vi "Que_Parse State.vi"(0 "State Queue":string, 7 "Error In (no error)":errorcluster) -> (4 "Remaining States":string, 6 "Current State":string, 8 "Arguments":string, 10 "PreState":string)   [LabVIEW 2016]
doc: "Parses the JKI State Machine state queue and returns the current state that will execute next with the associated arguments.\n\nFor instructions on how to use the JKI State Machine, examples and video tutorials, visit:\nhttp://jkisoft.com/state-machine/\n\n<B>Inputs:</B>\n <B>State Queue:</B> The entire state queue is wired to this input. This should come from the main JKI State Machine shift register.\n <B>Error In</B> The error cluster from the JKI State Machine is wired to this input. If an error occures and appears on this input, the current state output returns the \"Error Handler\" state.\n\n<B>Outputs:</B>\n <B>Remaining States:</B> Returns all the next states that should execute after the current state completes. These should be passed through the current state in the state machine. These can also be modified or augmented within the current state if necessary.\n <B>Current State:</B> Returns the current state that should execute next in the state machine. If an error is wired to the Error input then the current state output becomes \"Error Handler\".\n <B>Arguments:</B> Returns any argument(s) that may be used in the current state string. These arguments come after the \">>\" characters. <B>Note:</B> The arguments variable must not contain any unprintable characters like linefeed or carriage return.\n\n<B>State Syntax:</B>\nStateCategory: State >> Argument\nLine Terminator: Line feed\n <B>Example:</B>\nUI: Help >> About\n\nWhere \"UI\" is the state category\nWhere \"Help\" is the state\nWhere \"About\" is the argument\n <B>Other Examples:</B>\nApp Data: Initialize\nUI: Initialize\nHelp >> About\n\n<B>Commenting:</B>\nTo add a comment use \"//\" or \"#\" and all text to the right will be ignored\n <B>Commenting Example:</B>\nUI: Initialize // This initializes the UI\n# This whole line is a comment\n// Another comment line\n\nJKI State Machine™\nhttp://jkisoft.com/state-machine/\nCopyright (C) 2005-2008, JKI <info@jkisoft.com>\nALL RIGHTS RESERVED"
panel:
  # "For instructions on how to use the JKI State Machine, examples and video tutorials, visit:\nhttp://jkisoft.com/state-machine/\n\nJKI State Machine™\nhttp://jkisoft.com/state-machine/\nCopyright (C) 2005-2008, JKI <info@jkisoft.com>\nALL RIGHTS RESERVED"
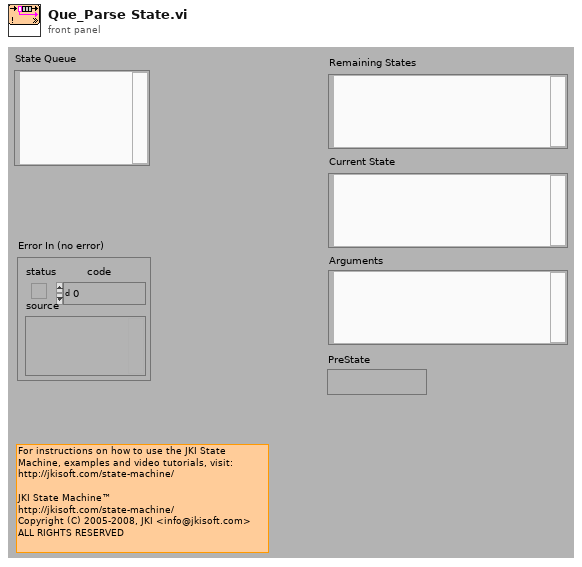
[diagram p1: front panel]
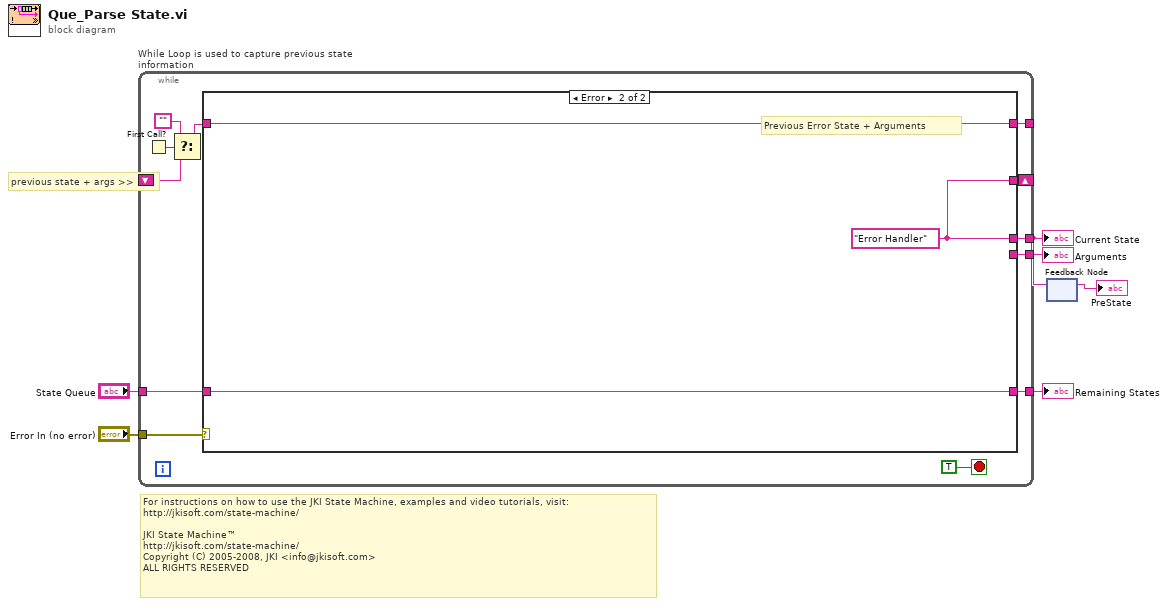
[diagram p0: block diagram]
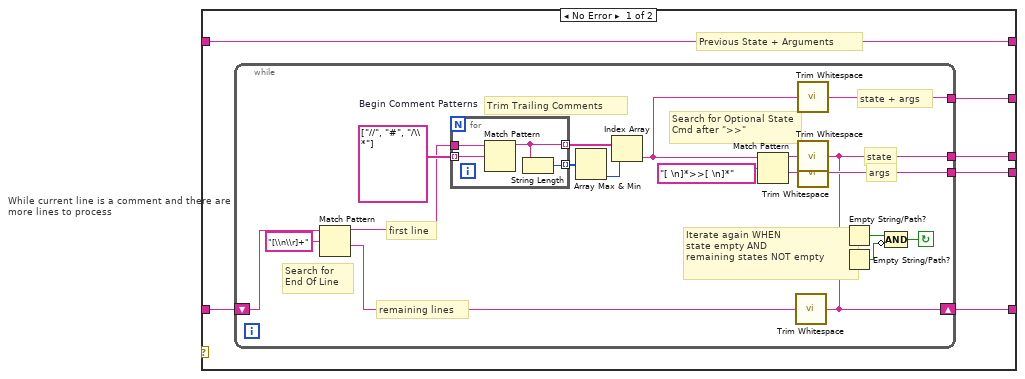
[diagram p2: hidden frame]
diagram:
  # "previous state + args >>"
  # "For instructions on how to use the JKI State Machine, examples and video tutorials, visit:\nhttp://jkisoft.com/state-machine/\n\nJKI State Machine™\nhttp://jkisoft.com/state-machine/\nCopyright (C) 2005-2008, JKI <info@jkisoft.com>\nALL RIGHTS RESERVED"
  n1 = while "While Loop is used to capture previous state information" {
    tunnel: [w18] -> w6
    tunnel: "State Queue" -> [w17]
    tunnel: "Error In (no error)" -> [w16]
    tunnel: [w15] -> w2
    tunnel: [w14] -> w3
    shift-right: [w12] -> _
    shift-left: _ -> [w10]
    tunnel: [w7] -> _
    stop <- TRUE stop-if-true
    n2 = First Call?() -> (First Call?: T/F=w11:bool)
    n3 = Select(t="", s=w11, f=w10) -> (s? t:f=w9:string)
    n4 = case shown="Error" w16 {
      tunnel: [w21 w50] -> w18
      tunnel: [w24 w48] -> w15
      tunnel: [w23 _] -> w14
      tunnel: w17 -> [w22 w50]
      tunnel: [w20 w48] -> w12
      tunnel: w9 -> [w19 w49]
      tunnel: [w19 w49] -> w7
      frame No Error {
        # "Previous State + Arguments"
        n5 = while "While current line is a comment and there are more lines to process" {
          tunnel: [w34] -> w24
          tunnel: [w35] -> w23
          shift-right: [w30] -> w21
          shift-left: w22 -> [w28]
          tunnel: [w25] -> w20
          stop <- w31 continue-if-true
          w42 = string[] ["//", "#", "/\\*"]  # Begin Comment Patterns
          # "state + args"
          # "remaining lines"
          # "first line"
          # "Search for End Of Line"
          # "Iterate again WHEN\nstate empty AND\nremaining states NOT empty"
          # "args"
          # "state"
          # "Search for Optional State Cmd after \">>\""
          # "Trim Trailing Comments"
          n6 = Match Pattern(string=w28, regular expression="[\\n\\r]+") -> (before substring=w27:string, after substring=w43:string)  [unwired: 3 out]
          n7 = for {
            tunnel: w27 -> [w47]
            tunnel: [w45] -> w39 mode=indexing
            tunnel: w42 -> [w46] mode=indexing
            tunnel: [w44] -> w41 mode=indexing
            n8 = Match Pattern(string=w47, regular expression=w46) -> (before substring=w45:string)  [unwired: 4 out]
            n9 = String Length(string=w45) -> (length=w44:i32)
          }
          n10 = Array Max & Min(array=w41) -> (min index (indices)=w40:i32)  [unwired: 3 out]
          n11 = Index Array(array=w39, index=w40) -> (element=w26:string)
          n12 = Match Pattern(string=w26, regular expression="[ \n]*>>[ \n]*") -> (before substring=w37:string, after substring=w36:string)  [unwired: 3 out]
          n13 = call <vilib>:"Trim Whitespace.vi"("string"=w43) -> ("trimmed string"=w30:string)  [unwired: 1 in]
          n14 = call <vilib>:"Trim Whitespace.vi"("string"=w26) -> ("trimmed string"=w25:string)  [unwired: 1 in]
          n15 = call <vilib>:"Trim Whitespace.vi"("string"=w37) -> ("trimmed string"=w34:string)  [unwired: 1 in]
          n16 = call <vilib>:"Trim Whitespace.vi"("string"=w36) -> ("trimmed string"=w35:string)  [unwired: 1 in]
          n17 = Empty String/Path?(string/path=w34) -> (empty?=w33:bool)
          n18 = Empty String/Path?(string/path=w30) -> (empty?=w32:bool)
          n19 = Compound Arithmetic op=AND(w33, invert w32) -> (w31:bool)
        }
      }
      frame Error {
        w48 = "Error Handler"
        # "Previous Error State + Arguments"
      }
    }
  }
  "Remaining States" <- w6
  "Arguments" <- w3
  "Current State" <- w2
  n20 = feedback-in #1(w2) -> ()
  n21 = feedback #1() -> (→"PreState":string)  [unwired: 1 in]
